vi "ReplaceObject.vi"(6 "name/order":string="LabVIEW Object In", 8 "error in (no error)":errorcluster, 11 "CreateInterface in":refnum<class "CreateInterface.lvclass">) -> (0 "error out":errorcluster)   [LabVIEW 2020, in "Mermaid.lvlib" / "CreateInterface.lvclass"]
uses:
  CreateInterface.lvclass
  CreateInterface.lvclass/CreateInterface.ctl
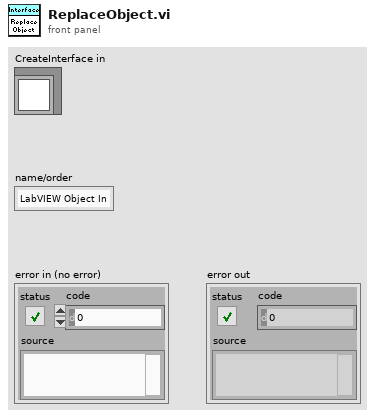
[diagram p1: front panel]
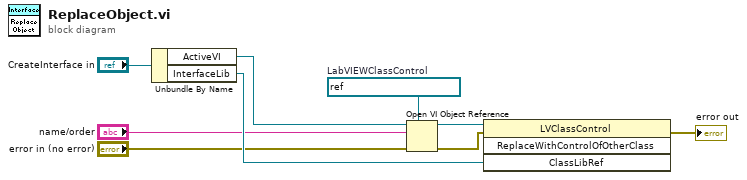
[diagram p0: block diagram]
diagram:
  w3 = refnum<vi> refnum  # LabVIEWClassControl
  n1 = Unbundle By Name("CreateInterface in") -> ("ActiveVI"=w8:refnum<vi>, "InterfaceLib"=w9:refnum<vi>)
  n2 = Open VI Object Reference(7:w3, 8:"error in (no error)", 10:"name/order", 11:w8) -> (0:w2:errorcluster, 3:w4:refnum<vi>)
  n3 = invoke class="LVClassControl" method="ReplaceWithControlOfOtherClass"(reference=w4, error in=w2, "ClassLibRef"=w9) -> (error out=→"error out":errorcluster)  [unwired: 1 in, 3 out]
